vi "DraggingDresser.vi"() -> ()   [LabVIEW 2014]
panel:
  out "Force":dbl[](array[numeric])
  out "Angle for Minimum Force":i32 format="%.1f"
  in  "Coefficient of Kinetic Friction":dbl format="%.1f"
  out "Waveform Graph":dbl[](graph)
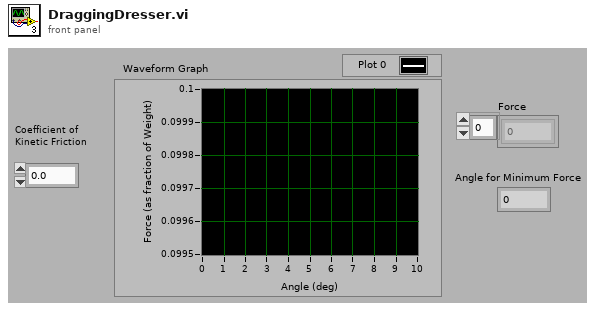
[diagram p1: front panel]
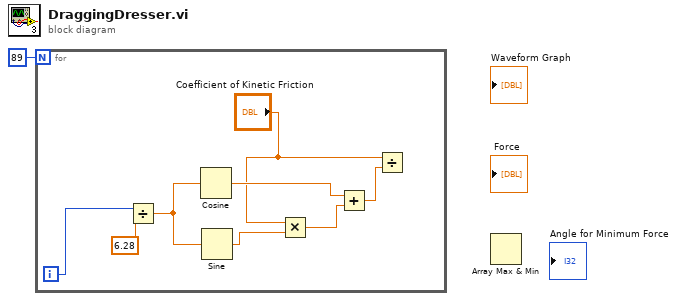
[diagram p0: block diagram]
diagram:
  n1 = for {
    N: 89 -> [_]
    i -> [w2]
    n2 = Divide(x=w2, y=6.28) -> (x/y=w4:dbl)
    n3 = Cosine(x=w4) -> (cos(x)=w9:dbl)
    n4 = Sine(x=w4) -> (sin(x)=w6:dbl)
    n5 = Multiply(x="Coefficient of Kinetic Friction", y=w6) -> (x*y=w5:dbl)
    n6 = Add(x=w9, y=w5) -> (x+y=w8:dbl)
    n7 = Divide(x="Coefficient of Kinetic Friction", y=w8) -> ()  [unwired: 1 out]
  }
  n8 = Array Max & Min() -> ()  [unwired: 1 in, 4 out]
